vi "InitDevice.vi"(8 "error in (no error)":errorcluster, 10 "address":string) -> (0 "error out":errorcluster, 1 "libraryVersion":string, 2 "connection":string, 3 "reference out":refnum<k7>)   [LabVIEW 2020]
panel:
  in  "Galil.IGalil":refnum<k7>
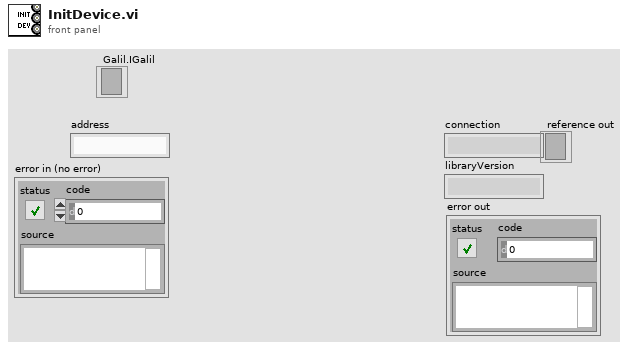
[diagram p1: front panel]
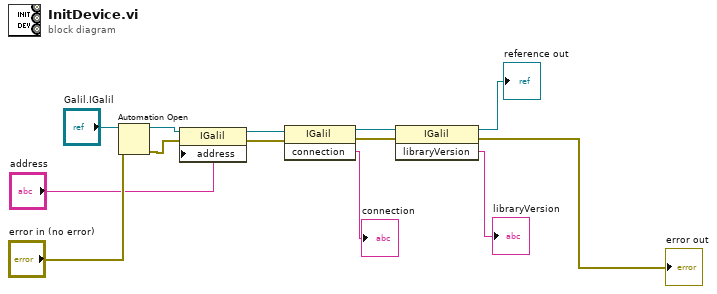
[diagram p0: block diagram]
diagram:
  n1 = Automation Open(error in (no error)="error in (no error)", Automation Refnum="Galil.IGalil") -> (Automation Refnum=w11:refnum<k7>, error out=w5:errorcluster)  [unwired: 2 in]
  n2 = property class="IGalil"(reference=w11, error in=w5, "address"="address") -> (reference out=w9:refnum<k7>, error out=w4:errorcluster)
  n3 = invoke class="IGalil" method="connection"(reference=w9, error in=w4) -> (reference out=w7:refnum<k7>, error out=w3:errorcluster, "connection"=→"connection":string)  [unwired: 1 in]
  n4 = invoke class="IGalil" method="libraryVersion"(reference=w7, error in=w3) -> (reference out=→"reference out":refnum<k7>, error out=→"error out":errorcluster, "libraryVersion"=→"libraryVersion":string)  [unwired: 1 in]
